vi "SIM Runge-Kutta embedded int (array).vi"(3 "Simulation data":T1={"continuous integrator"=enum."RK 1 (Euler)", "initial time"=0.1, "final time"=4.0, "step size"=600.0, "proposed step size"=1e-07, "max step size"=0.001, "min step size"=0.0, "discrete time step"=0.0, "max step ratio"=3.0, "Diag Eval Stage"=enum."Major Substep", "Substep Index"=0, "Timestep Index"=10.0, "simulation time"=0.0, "current timestep base"=0.01, "proposed step time"=0.0, "absolute tolerance"=0.0, "relative tolerance"=0.0, "step accepted?"=FALSE, "step complete?"=FALSE, "Halt?"=FALSE, "reset integrator?"=FALSE, "machine epsilon"=6.0, "min float"=0.0, "error"={"status"=FALSE, "code"=0, "source"=""}, "Method Order"=0, "Finished Late [i-1]"=FALSE, "Discrete step?"=FALSE, "NaN and Inf check?"=FALSE, "Final Timestep Index"=0.0, "(maj+disc)or(init)?"=FALSE, "Full Solver Reset"=TRUE, "Execution Mode"=0, "check vector sizes?"=FALSE, "solver handles zc?"=FALSE, "Simulation Registry"={"Current Idx"=0, "Node Tags"=[], "Node Headers"=[], "Node Data"=[], "Cont State data"={"inputs"=[], "outputs"=[], "reset"=[], "lower limits"=[], "upper limits"=[], "limit types"=[], "reset types"=[], "initial conditions"=[], "reset I.C."=[], "limited?"=[], "State Names"=[]}, "DiscreteInfo"={"tick period (sec)"=0.0, "time (ticks)"=0, "fire?"=[], "registry"={"period (sec)"=[], "skew (sec)"=[], "period (tick)"=[], "skew (tick)"=[]}, "discrete \nblocks?"=FALSE, "steps per tick"=0.0, "steps to tick"=0.0, "discrete \ntick?"=FALSE}, "Disc State data"={"Disc States"=[], "State Names"=[]}, "Registry Error"={"Error Block ID"=0, "code"=0}, "ZC Indices"=[]}, "variable step solver?"=FALSE, "First Substep?"=FALSE, "Continuous States?"=FALSE} {"Execution Mode" items=["Simulate to Completion", "Single Time-Step Simulation (Fixed Step Only)"]; "min float" format="%.1e"; "proposed step size" format="%.1e"; "proposed step time" format="%.1e"; "max step ratio" format="%.1e"; "min step size" format="%.1e"; "machine epsilon" format="%.1e"; "discrete time step" format="%.1e"; "max step size" format="%.1e"; "current timestep base" format="%.1e"; "final time" format="%.1e"; "simulation time" format="%.1e"; "relative tolerance" format="%.1e"; "absolute tolerance" format="%.1e"; "Substep Index" format="%.1e"; "step size" format="%.1e"; "initial time" format="%.1e"}) -> (1 "Simulation data out":T1={"continuous integrator"=enum."RK 1 (Euler)", "initial time"=0.1, "final time"=4.0, "step size"=600.0, "proposed step size"=1e-07, "max step size"=0.001, "min step size"=0.0, "discrete time step"=0.0, "max step ratio"=3.0, "Diag Eval Stage"=enum."Major Substep", "Substep Index"=0, "Timestep Index"=10.0, "simulation time"=0.0, "current timestep base"=0.01, "proposed step time"=0.0, "absolute tolerance"=0.0, "relative tolerance"=0.0, "step accepted?"=FALSE, "step complete?"=FALSE, "Halt?"=FALSE, "reset integrator?"=FALSE, "machine epsilon"=6.0, "min float"=0.0, "error"={"status"=FALSE, "code"=0, "source"=""}, "Method Order"=0, "Finished Late [i-1]"=FALSE, "Discrete step?"=FALSE, "NaN and Inf check?"=FALSE, "Final Timestep Index"=0.0, "(maj+disc)or(init)?"=FALSE, "Full Solver Reset"=TRUE, "Execution Mode"=0, "check vector sizes?"=FALSE, "solver handles zc?"=FALSE, "Simulation Registry"={"Current Idx"=0, "Node Tags"=[], "Node Headers"=[], "Node Data"=[], "Cont State data"={"inputs"=[], "outputs"=[], "reset"=[], "lower limits"=[], "upper limits"=[], "limit types"=[], "reset types"=[], "initial conditions"=[], "reset I.C."=[], "limited?"=[], "State Names"=[]}, "DiscreteInfo"={"tick period (sec)"=0.0, "time (ticks)"=0, "fire?"=[], "registry"={"period (sec)"=[], "skew (sec)"=[], "period (tick)"=[], "skew (tick)"=[]}, "discrete \nblocks?"=FALSE, "steps per tick"=0.0, "steps to tick"=0.0, "discrete \ntick?"=FALSE}, "Disc State data"={"Disc States"=[], "State Names"=[]}, "Registry Error"={"Error Block ID"=0, "code"=0}, "ZC Indices"=[]}, "variable step solver?"=FALSE, "First Substep?"=FALSE, "Continuous States?"=FALSE} {"Execution Mode" items=["Simulate to Completion", "Single Time-Step Simulation (Fixed Step Only)"]; "min float" format="%.1e"; "proposed step size" format="%.1e"; "proposed step time" format="%.1e"; "max step ratio" format="%.1e"; "min step size" format="%.1e"; "machine epsilon" format="%.1e"; "discrete time step" format="%.1e"; "max step size" format="%.1e"; "current timestep base" format="%.1e"; "final time" format="%.1e"; "simulation time" format="%.1e"; "relative tolerance" format="%.1e"; "absolute tolerance" format="%.1e"; "Substep Index" format="%.1e"; "step size" format="%.1e"; "initial time" format="%.1e"})   [LabVIEW 2010]
uses:
  SIM simulation data.ctl
  SIM integration method.ctl
  SIM diagram eval stage.ctl
  SIMSCR Execution Mode.ctl
  SIM Simulation Registry.ctl
  SIM Registry Node Header.ctl
  SIM Registry Node Record.ctl
  SIM trigger type.ctl
  SIM solver state data.ctl
  SIM limit type.ctl
  SIM discrete data.ctl
  SIM Discrete state data.ctl
  SIM Simulation Registry Error.ctl
  SIM limit signal (array).vi
panel:
  # "General Runge-Kutta integrator of order s.\n\nSolves the initial value problem \n\ny'(t) = f(t,y)\n\nby propogating the solution from y(t_n) to y(t_(n+1)), using the intermediate function evaluations k_i. The stepsize is defined as h = t_(n+1) - t_n.\n\nk_i = f( t_n + c_i h, y_n + h sum(j = 1 to s)(a_ij k_j) ) (1 <= i <= s)\n\ny_(n+1) = y_n + h sum(j = 1 to s)(a_(s-1)j k_j )\n\nNOTE This VI is paired with a time advancer that makes the simulation time appropriate for evaluating the k_i.\n\nNOTE This implementation assumes that c_0 = 0 and that\na_0j = 0 for a <= j <= s. The first row (all zeros) of the matrix a\nis omitted, and the last row of a stores the coefficients for the final output. Consequently, in the equation for k_i, a_ij should really read a_(i-1)j ."
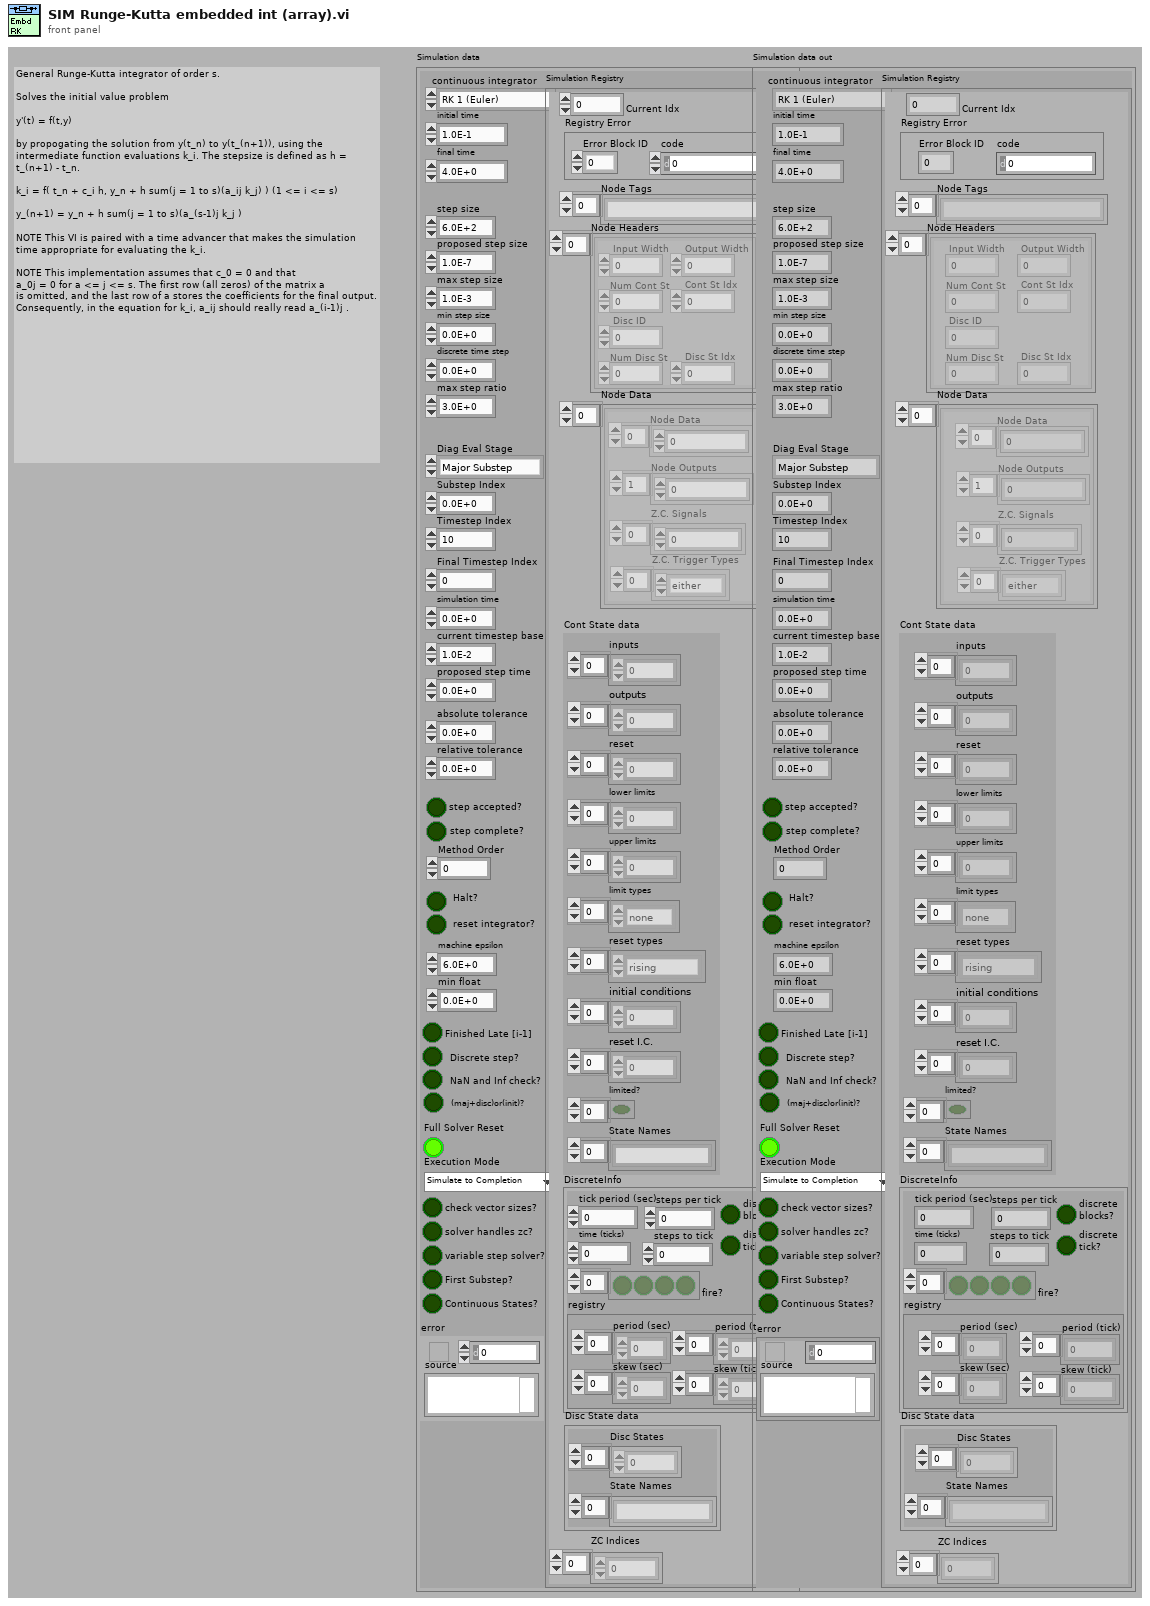
[diagram p1: front panel]
types:
  T1 = typedef "SIM simulation data.ctl" = cluster{"continuous integrator":T2, "initial time":dbl, "final time":dbl, "step size":dbl, "proposed step size":dbl, "max step size":dbl, "min step size":dbl, "discrete time step":dbl, "max step ratio":dbl, "Diag Eval Stage":T3, "Substep Index":i32, "Timestep Index":dbl, "simulation time":dbl, "current timestep base":dbl, "proposed step time":dbl, "absolute tolerance":dbl, "relative tolerance":dbl, "step accepted?":bool, "step complete?":bool, "Halt?":bool, "reset integrator?":bool, "machine epsilon":dbl, "min float":dbl, "error":errorcluster, "Method Order":u32, "Finished Late [i-1]":bool, "Discrete step?":bool, "NaN and Inf check?":bool, "Final Timestep Index":dbl, "(maj+disc)or(init)?":bool, "Full Solver Reset":bool, "Execution Mode":T4, "check vector sizes?":bool, "solver handles zc?":bool, "Simulation Registry":T5, "variable step solver?":bool, "First Substep?":bool, "Continuous States?":bool}
  T2 = typedef "SIM integration method.ctl" = enum16{"RK 1 (Euler)", "Linearizer", "State Query", "Trim Eval", "Adams", "RK 3", "RK 4", "RK 45", "BDF", "RK 2", "RK 23", "Rosenbrock", "Discrete States Only"}
  T3 = typedef "SIM diagram eval stage.ctl" = enum16{"Init", "Minor Substep", "Major Substep", "Final"}
  T4 = typedef "SIMSCR Execution Mode.ctl" = u16
  T5 = typedef "SIM Simulation Registry.ctl" = cluster{"Current Idx":i32, "Node Tags":string[], "Node Headers":T6[], "Node Data":T7[], "Cont State data":T9, "DiscreteInfo":T11, "Disc State data":T12, "Registry Error":T13, "ZC Indices":i32[]}
  T6 = typedef "SIM Registry Node Header.ctl" = cluster{"Input Width":i32, "Disc ID":i32, "Num Cont St":i32, "Cont St Idx":i32, "Num Disc St":i32, "Disc St Idx":i32, "Output Width":i32}
  T7 = typedef "SIM Registry Node Record.ctl" = cluster{"Node Data":dbl[], "Node Outputs":dbl[], "Z.C. Signals":dbl[], "Z.C. Trigger Types":T8[]}
  T8 = typedef "SIM trigger type.ctl" = enum16{"rising", "falling", "either", "none"}
  T9 = typedef "SIM solver state data.ctl" = cluster{"inputs":dbl[], "outputs":dbl[], "reset":dbl[], "lower limits":dbl[], "upper limits":dbl[], "limit types":T10[], "reset types":T8[], "initial conditions":dbl[], "reset I.C.":dbl[], "limited?":bool[], "State Names":string[]}
  T10 = typedef "SIM limit type.ctl" = enum16{"upper", "lower", "both", "none"}
  T11 = typedef "SIM discrete data.ctl" = cluster{"tick period (sec)":dbl, "time (ticks)":i32, "fire?":bool[], "registry":cluster{"period (sec)":dbl[], "skew (sec)":dbl[], "period (tick)":i32[], "skew (tick)":i32[]}, "discrete \nblocks?":bool, "steps per tick":dbl, "steps to tick":dbl, "discrete \ntick?":bool}
  T12 = typedef "SIM Discrete state data.ctl" = cluster{"Disc States":dbl[], "State Names":string[]}
  T13 = typedef "SIM Simulation Registry Error.ctl" = cluster{"Error Block ID":i32, "code":i32}
  T14 = typedef "SIM Runga-Kutte data - variable step.ctl" = cluster{"weighting coefficients":dbl[][], "time step fractions":dbl[], "Number of sub steps":i32, "error coefficients":dbl[], "error order":i32}
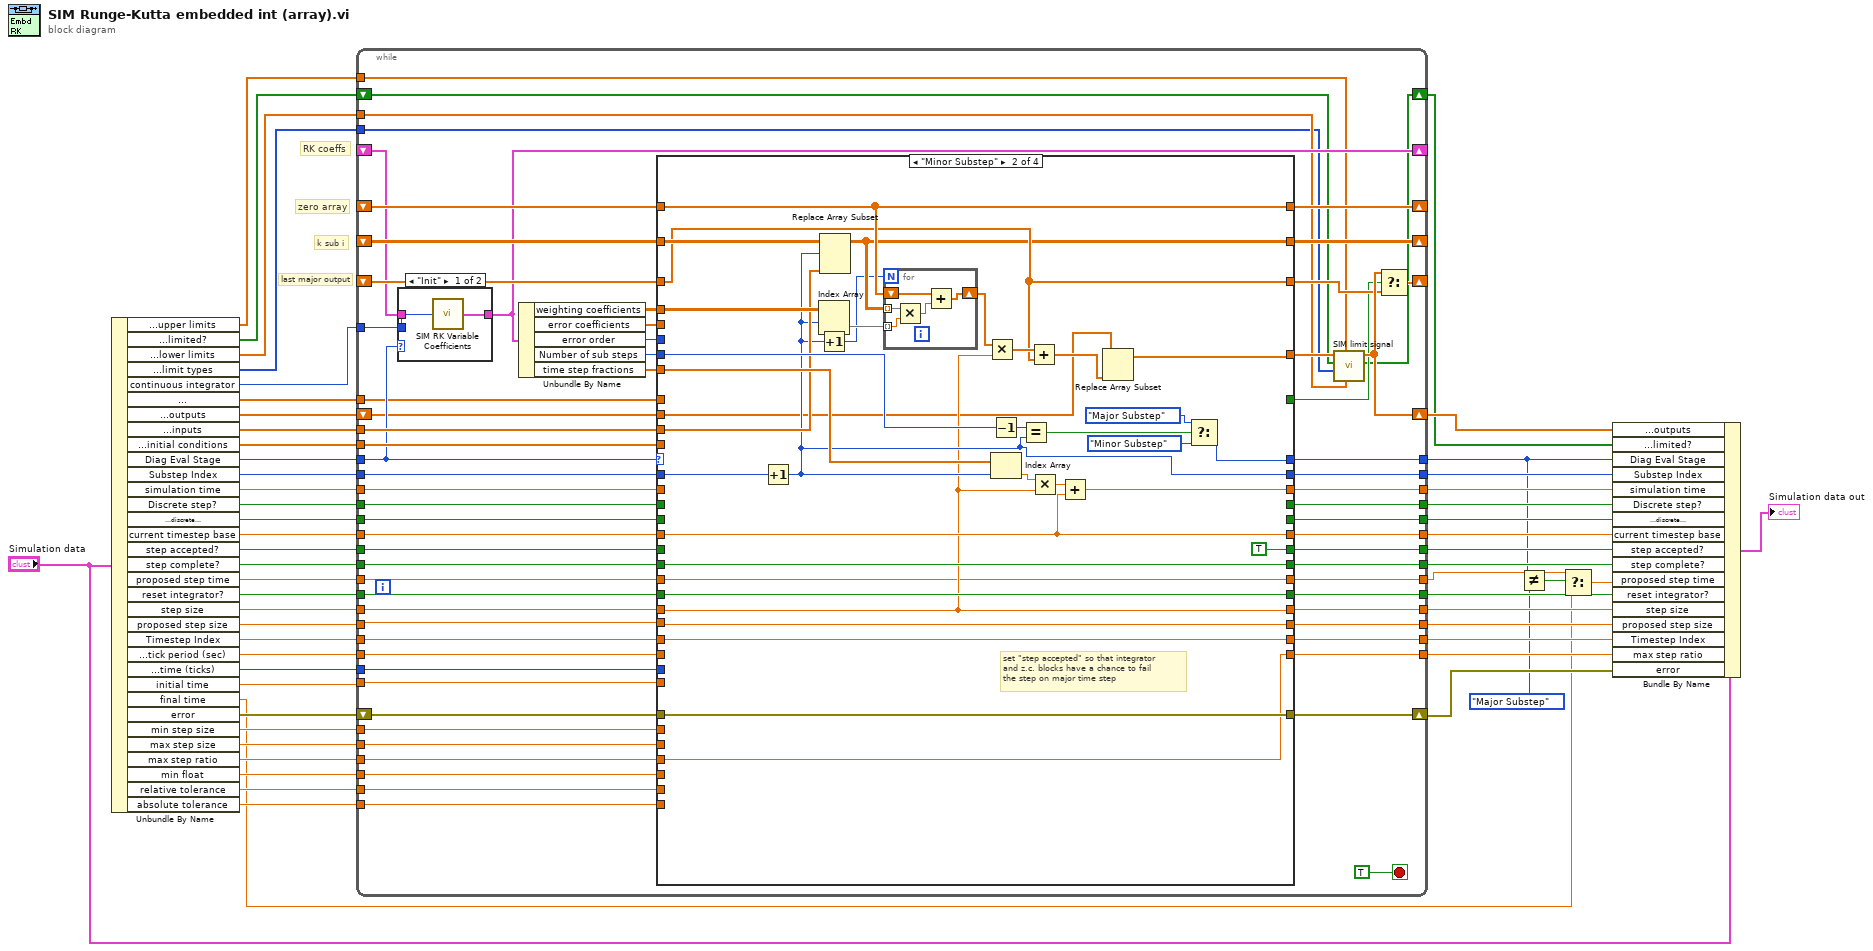
[diagram p0: block diagram]
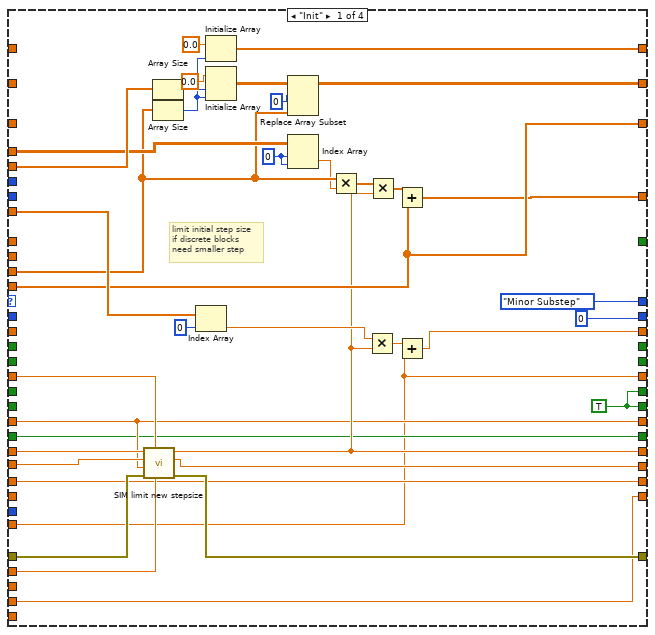
[diagram p3: hidden frame]
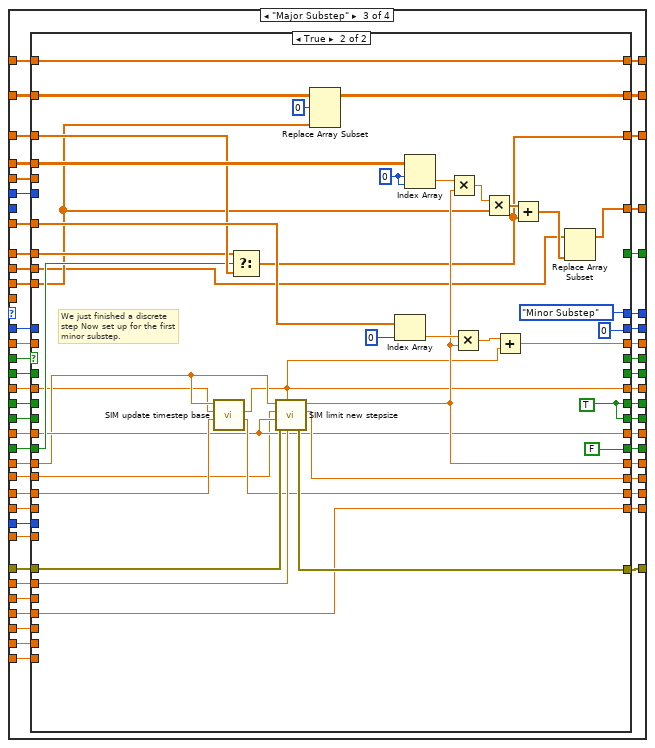
[diagram p4: hidden frame]
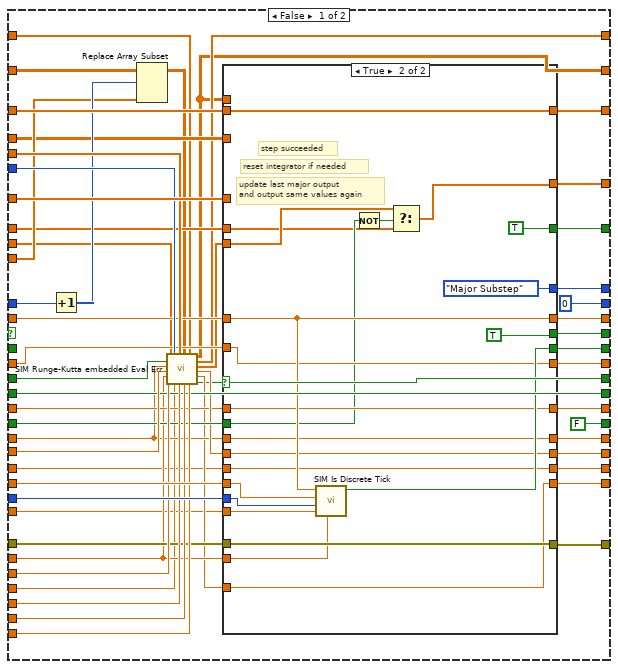
[diagram p5: hidden frame]
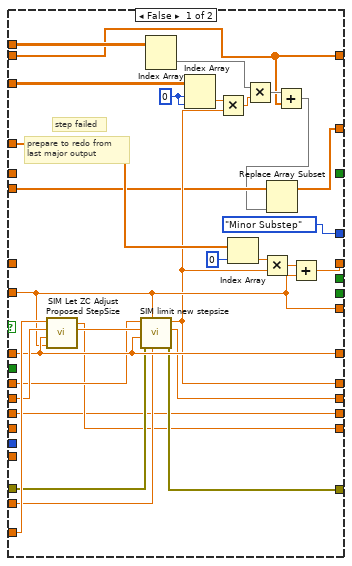
[diagram p6: hidden frame]
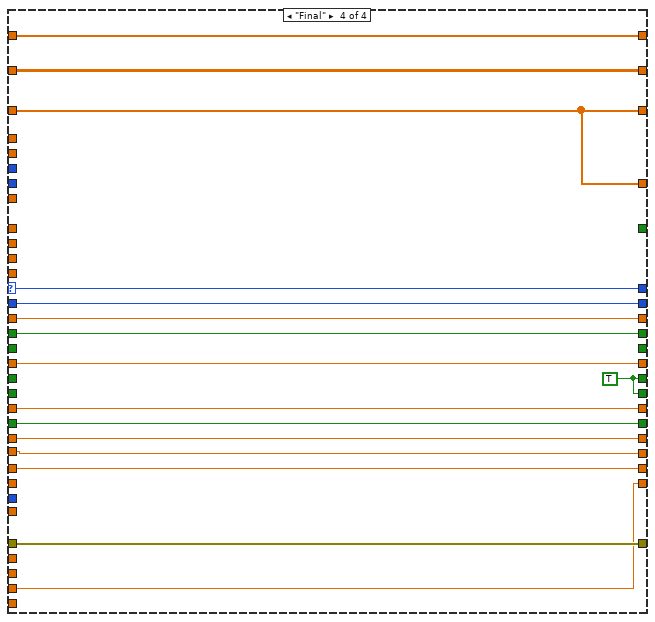
[diagram p7: hidden frame]
diagram:
  # "RK coeffs"
  # "last major output"
  # "k sub i"
  # "zero array"
  n1 = Unbundle By Name("Simulation data") -> ("Simulation Registry.Cont State data.upper limits"=w13:dbl[], "Simulation Registry.Cont State data.limited?"=w10:bool[], "Simulation Registry.Cont State data.lower limits"=w12:dbl[], "Simulation Registry.Cont State data.limit types"=w11:T10[], "continuous integrator"=w32:T2, "Simulation Registry.Cont State data.reset I.C."=w16:dbl[], "Simulation Registry.Cont State data.outputs"=w15:dbl[], "Simulation Registry.Cont State data.inputs"=w42:dbl[], "Simulation Registry.Cont State data.initial conditions"=w41:dbl[], "Diag Eval Stage"=w43:T3, "Substep Index"=w44:i32, "simulation time"=w38:dbl, "Discrete step?"=w8:bool, "Simulation Registry.DiscreteInfo.discrete \ntick?"=w7:bool, "current timestep base"=w36:dbl, "step accepted?"=w17:bool, "step complete?"=w27:bool, "proposed step time"=w35:dbl, "reset integrator?"=w29:bool, "step size"=w31:dbl, "proposed step size"=w30:dbl, "Timestep Index"=w23:dbl, "Simulation Registry.DiscreteInfo.tick period (sec)"=w40:dbl, "Simulation Registry.DiscreteInfo.time (ticks)"=w39:i32, "initial time"=w37:dbl, "final time"=w2:dbl, "error"=w28:errorcluster, "min step size"=w24:dbl, "max step size"=w22:dbl, "max step ratio"=w21:dbl, "min float"=w20:dbl, "relative tolerance"=w19:dbl, "absolute tolerance"=w18:dbl)
  n2 = while {
    shift-right: [w111] -> _
    shift-left: _ -> [w119]
    tunnel: w11 -> [w102]
    tunnel: w12 -> [w103]
    tunnel: w13 -> [w104]
    shift-right: [w110] -> _
    shift-left: _ -> [w115]
    shift-right: [w117] -> _
    shift-left: _ -> [w118]
    shift-right: [w106] -> _
    shift-left: _ -> [w105]
    tunnel: [w101] -> w5
    tunnel: [w100] -> w53
    tunnel: [w99] -> w52
    tunnel: [w98] -> w51
    tunnel: [w97] -> w50
    tunnel: [w96] -> w49
    tunnel: [w95] -> w48
    tunnel: [w94] -> w47
    tunnel: [w93] -> w3
    tunnel: [w92] -> w46
    tunnel: w44 -> [w91]
    tunnel: w43 -> [w88]
    tunnel: w42 -> [w90]
    tunnel: w41 -> [w89]
    tunnel: w8 -> [w87]
    tunnel: w40 -> [w86]
    tunnel: w39 -> [w85]
    tunnel: w38 -> [w84]
    tunnel: w37 -> [w82]
    tunnel: w36 -> [w81]
    tunnel: w24 -> [w78]
    tunnel: w35 -> [w77]
    tunnel: [w76] -> w34
    tunnel: [w75] -> w33
    tunnel: w32 -> [w74]
    tunnel: w31 -> [w73]
    tunnel: w30 -> [w72]
    tunnel: w29 -> [w71]
    tunnel: w27 -> [w70]
    tunnel: w23 -> [w69]
    tunnel: [w68] -> w25
    tunnel: w22 -> [w67]
    tunnel: w21 -> [w66]
    tunnel: w20 -> [w65]
    tunnel: w19 -> [w64]
    tunnel: w18 -> [w63]
    tunnel: w17 -> [w62]
    tunnel: w16 -> [w61]
    tunnel: [w59] -> w14
    shift-right: [w57] -> w9
    shift-left: w10 -> [w58]
    shift-right: [w109] -> w55
    shift-left: w15 -> [w60]
    shift-right: [w79] -> w26
    shift-left: w28 -> [w80]
    tunnel: w7 -> [w56]
    stop <- TRUE stop-if-true
    n3 = case shown="\"Init\"" w88 {
      tunnel: [w123 w124] -> w106
      tunnel: w105 -> [_ w124]
      tunnel: w74 -> [w122 _]
      frame "Init" {
        n4 = call "SIM RK Variable Coefficients.vi"("continuous integrator"=w122) -> ("Runga-Kutte data"=w123:T14)
      }
      frame Default {
      }
    }
    n5 = Unbundle By Name(w106) -> ("weighting coefficients"=w83:dbl[][], "error coefficients"=w114:dbl[], "error order"=w113:i32, "Number of sub steps"=w121:i32, "time step fractions"=w120:dbl[])
    n6 = case shown="\"Minor Substep\"" w88 {
      selector: w88 -> [_ _ _ w412]
      tunnel: [0 w177 w254 w411] -> w100
      tunnel: w120 -> [w161 w197 w252 _]
      tunnel: [w157 w194 w253 w408] -> w99
      tunnel: [SIM_diagram_eval_stage."Minor Substep" ("Diagram Eval Stage") w190 w251 w412] -> w101
      tunnel: w121 -> [_ w193 _ _]
      tunnel: w119 -> [_ w187 w244 w415]
      tunnel: w118 -> [_ w183 w250 w414]
      tunnel: w89 -> [w143 _ _ _]
      tunnel: [w147 w180 w240 w415] -> w111
      tunnel: [w151 w183 w238 w414] -> w117
      tunnel: w114 -> [w150 _ w248 _]
      tunnel: w115 -> [_ w181 w247 w413]
      tunnel: [w143 w181 w246 w413] -> w108
      tunnel: w91 -> [_ w178 w245 w411]
      tunnel: w113 -> [_ _ w249 _]
      tunnel: w90 -> [w127 w179 w243 _]
      tunnel: w83 -> [w141 w186 w241 _]
      tunnel: [w142 w165 w242 w413] -> w112
      tunnel: [_ _ w239 _] -> w107
      tunnel: w87 -> [_ _ w237 w410]
      tunnel: [_ _ w236 w410] -> w98
      tunnel: w85 -> [_ _ w235 _]
      tunnel: w86 -> [_ _ w234 _]
      tunnel: [_ _ w233 _] -> w97
      tunnel: [w125 w174 w216 w407] -> w96
      tunnel: [w140 TRUE ("step accepted?") w231 w409] -> w95
      tunnel: [w140 w173 w230 w409] -> w94
      tunnel: [w131 w163 w217 w406] -> w93
      tunnel: [w130 w172 w232 w405] -> w92
      tunnel: w84 -> [_ _ w207 w408]
      tunnel: w73 -> [w134 w171 w209 w404]
      tunnel: w82 -> [w125 _ w203 _]
      tunnel: w81 -> [w139 w174 w227 w407]
      tunnel: w80 -> [w138 w169 w221 w402]
      tunnel: [w137 w169 w222 w402] -> w79
      tunnel: w78 -> [w136 _ w223 _]
      tunnel: w72 -> [w135 w170 w225 w403]
      tunnel: w77 -> [w131 w163 w224 w406]
      tunnel: [w133 w171 w219 w404] -> w76
      tunnel: [w132 w170 w220 w403] -> w75
      tunnel: w71 -> [w130 w172 w228 w405]
      tunnel: w70 -> [_ w173 w206 _]
      tunnel: w61 -> [_ _ w229 _]
      tunnel: w69 -> [w129 w168 w226 w400]
      tunnel: [w129 w168 w218 w400] -> w68
      tunnel: w67 -> [_ _ w215 _]
      tunnel: w66 -> [w128 w167 w214 w401]
      tunnel: w65 -> [_ _ w213 _]
      tunnel: w64 -> [_ _ w212 _]
      tunnel: w63 -> [_ _ w211 _]
      tunnel: w62 -> [_ _ w210 _]
      tunnel: w60 -> [_ w164 w208 _]
      tunnel: [w128 w167 w205 w401] -> w59
      tunnel: w56 -> [_ _ w204 _]
      frame "Init" {
        w146 = 0 ("index (row)")
        w140 = TRUE ("step accepted?")
        # "limit initial step size\nif discrete blocks\nneed smaller step"
        n7 = call "SIM limit new stepsize.vi"("min step size"=w136, "current timestep base"=w139, "error"=w138, "proposed step time"=w131, "proposed step size"=w135, "step size"=w134) -> ("error out"=w137:errorcluster, "proposed step size"=w132:dbl, "step size"=w133:dbl)  [unwired: 1 in, 2 out]
        n8 = Array Size(array=w150) -> (size(s)=w155:i32)
        n9 = Array Size(array=w127) -> (size(s)=w152:i32)
        n10 = Index Array(array=w161, index=0) -> (element=w159:dbl)
        n11 = Initialize Array(0.0 ("element"), w152) -> (w151:dbl[])
        n12 = Initialize Array(0.0 ("element"), w155, w152) -> (w149:dbl[][])
        n13 = Replace Array Subset(array=w149, new element=w127, index (row)=0) -> (w147:dbl[][])  [unwired: 1 in]
        n14 = Index Array(array=w141, index (row)=w146, index (col)=w146) -> (element=w126:dbl)
        n15 = Multiply(x=w127, y=w126) -> (x*y=w145:dbl[])
        n16 = Multiply(x=w159, y=w133) -> (x*y=w158:dbl)
        n17 = Multiply(x=w145, y=w133) -> (x*y=w144:dbl[])
        n18 = Add(x=w144, y=w143) -> (x+y=w142:dbl[])
        n19 = Add(x=w158, y=w125) -> (x+y=w157:dbl)
      }
      frame "Minor Substep" {
        # "set \"step accepted\" so that integrator\nand z.c. blocks have a chance to fail \nthe step on major time step"
        n20 = Increment(x=w178) -> (x+1=w177:i32)
        n21 = Index Array(array=w186, index (row)=w177) -> (element=w184:dbl[])  [unwired: 1 in]
        n22 = Increment(x=w177) -> (x+1=w176:i32)
        n23 = Replace Array Subset(array=w187, new element=w179, index (row)=w177) -> (w180:dbl[][])  [unwired: 1 in]
        n24 = for {
          N: w176 -> [_]
          tunnel: w180 -> [w202] mode=indexing
          tunnel: w184 -> [w201] mode=indexing
          shift-right: [w199] -> w185
          shift-left: w183 -> [w198]
          n25 = Multiply(x=w202, y=w201) -> (x*y=w200:dbl[])
          n26 = Add(x=w198, y=w200) -> (x+y=w199:dbl[])
        }
        n27 = Multiply(x=w185, y=w171) -> (x*y=w182:dbl[])
        n28 = Decrement(x=w193) -> (x-1=w192:i32)
        n29 = Index Array(array=w197, index=w177) -> (element=w196:dbl)
        n30 = Equal?(x=w192, y=w177) -> (x = y?=w191:bool)
        n31 = Add(x=w182, y=w181) -> (x+y=w166:dbl[])
        n32 = Multiply(x=w196, y=w171) -> (x*y=w195:dbl)
        n33 = Add(x=w195, y=w174) -> (x+y=w194:dbl)
        n34 = Replace Array Subset(array=w164, new element=w166) -> (w165:dbl[])  [unwired: 1 in]
        n35 = Select(t=SIM_diagram_eval_stage."Major Substep" ("Diagram Eval Stage"), s=w191, f=SIM_diagram_eval_stage."Minor Substep" ("Diagram Eval Stage")) -> (s? t:f=w190:T3)
      }
      frame "Major Substep" {
        n36 = case shown="True" w237 {
          tunnel: [0 ("Substep Index") 0 ("Substep Index")] -> w254
          tunnel: [w307 w365] -> w253
          tunnel: w252 -> [w306 w385]
          tunnel: [w305 SIM_diagram_eval_stage."Minor Substep" ("Diagram Eval Stage")] -> w251
          tunnel: w250 -> [w262 w389]
          tunnel: w249 -> [w304 _]
          tunnel: w248 -> [w303 _]
          tunnel: w247 -> [w302 w384]
          tunnel: [w301 w370] -> w246
          tunnel: w245 -> [w300 _]
          tunnel: w244 -> [w299 w390]
          tunnel: w243 -> [w297 w372]
          tunnel: [w296 w366] -> w242
          tunnel: w241 -> [w295 w391]
          tunnel: [w257 w388] -> w240
          tunnel: [w294 _] -> w239
          tunnel: [w261 w389] -> w238
          tunnel: [w293 _] -> w236
          tunnel: w235 -> [w292 _]
          tunnel: w234 -> [w291 _]
          tunnel: [w290 _] -> w233
          tunnel: [FALSE ("reset integrator?") FALSE ("reset integrator?")] -> w232
          tunnel: [w260 w383] -> w231
          tunnel: [w280 w383] -> w230
          tunnel: w229 -> [w283 w382]
          tunnel: w228 -> [w282 w381]
          tunnel: w227 -> [w278 w362]
          tunnel: w226 -> [w265 w379]
          tunnel: w225 -> [w284 w363]
          tunnel: w224 -> [w275 w371]
          tunnel: w223 -> [w271 w378]
          tunnel: [w272 w377] -> w222
          tunnel: w221 -> [w273 w376]
          tunnel: [w276 w375] -> w220
          tunnel: [w266 w374] -> w219
          tunnel: [w264 w373] -> w218
          tunnel: [w274 w371] -> w217
          tunnel: [w267 w361] -> w216
          tunnel: w215 -> [w288 _]
          tunnel: w214 -> [w269 w369]
          tunnel: w213 -> [w287 _]
          tunnel: w212 -> [w286 _]
          tunnel: w211 -> [w285 _]
          tunnel: w210 -> [w279 _]
          tunnel: w209 -> [w270 w364]
          tunnel: w208 -> [w259 w367]
          tunnel: w207 -> [w281 _]
          tunnel: w206 -> [w280 _]
          tunnel: [w256 w369] -> w205
          tunnel: w204 -> [_ _]
          tunnel: w203 -> [w255 _]
          frame False {
            n37 = Increment(x=w300) -> (x+1=w298:i32)
            n38 = Replace Array Subset(array=w299, new element=w297, index (row)=w298) -> (w263:dbl[][])  [unwired: 1 in]
            n39 = call "SIM Runge-Kutta embedded Eval Err.vi"("outputs"=w259, "step accepted?"=w279, "step size"=w270, "proposed step size"=w284, "min step size"=w271, "max step size"=w288, "error order"=w304, "max step ratio"=w269, "error coefficients"=w303, "min float"=w287, "k sub i"=w263, "relative tolerance"=w286, "Zero Array"=w262, "absolute tolerance"=w285) -> ("k sub i out"=w257:dbl[][], "Zero Array Out"=w261:dbl[], "outputs out"=w258:dbl[], "proposed step size out"=w277:dbl, "new step size ratio"=w268:dbl, "step accepted? out"=w260:bool)
            n40 = case shown="True" w260 {
              tunnel: [w338 w353] -> w307
              tunnel: w306 -> [w337 _]
              tunnel: [SIM_diagram_eval_stage."Minor Substep" ("Diagram Eval Stage") SIM_diagram_eval_stage."Major Substep" ("Diagram Eval Stage")] -> w305
              tunnel: w302 -> [w309 w359]
              tunnel: [w309 w359] -> w301
              tunnel: [w313 w357] -> w296
              tunnel: w257 -> [w330 _]
              tunnel: w295 -> [w331 _]
              tunnel: [_ TRUE] -> w294
              tunnel: [_ TRUE] -> w293
              tunnel: w292 -> [_ w355]
              tunnel: w291 -> [_ w350]
              tunnel: [_ w354] -> w290
              tunnel: w283 -> [_ w341]
              tunnel: w282 -> [_ w343]
              tunnel: w258 -> [w315 w342]
              tunnel: w281 -> [_ w353]
              tunnel: w268 -> [w326 w348]
              tunnel: w278 -> [w317 w347]
              tunnel: w277 -> [w325 w351]
              tunnel: [w311 w351] -> w276
              tunnel: w275 -> [w323 w352]
              tunnel: [w323 w352] -> w274
              tunnel: w273 -> [w322 w349]
              tunnel: [w321 w349] -> w272
              tunnel: w271 -> [w320 w339]
              tunnel: w270 -> [w319 w345]
              tunnel: [w318 w348] -> w256
              tunnel: [w317 w347] -> w267
              tunnel: [w316 w345] -> w266
              tunnel: w265 -> [w310 w346]
              tunnel: [w310 w346] -> w264
              tunnel: w255 -> [_ w340]
              frame False {
                w333 = 0 ("index (row)")
                # "step failed"
                # "prepare to redo from\nlast major output"
                n41 = call "SIM Let ZC Adjust Proposed StepSize.vi"("current timestep base"=w317, "proposed step time"=w323, "proposed step size"=w325, "max step ratio"=w326) -> ("proposed step size out"=w324:dbl, "max step ratio out"=w318:dbl)  [unwired: 2 out]
                n42 = call "SIM limit new stepsize.vi"("min step size"=w320, "current timestep base"=w317, "error"=w322, "proposed step time"=w323, "proposed step size"=w324, "step size"=w319) -> ("error out"=w321:errorcluster, "proposed step size"=w311:dbl, "step size"=w316:dbl)  [unwired: 1 in, 2 out]
                n43 = Index Array(array=w330) -> (element=w327:dbl[])  [unwired: 2 in]
                n44 = Index Array(array=w331, index (row)=w333, index (col)=w333) -> (element=w329:dbl)
                n45 = Multiply(x=w329, y=w316) -> (x*y=w328:dbl)
                n46 = Index Array(array=w337, index=0) -> (element=w336:dbl)
                n47 = Multiply(x=w327, y=w328) -> (x*y=w332:dbl[])
                n48 = Multiply(x=w336, y=w316) -> (x*y=w334:dbl)
                n49 = Add(x=w332, y=w309) -> (x+y=w314:dbl[])
                n50 = Replace Array Subset(array=w315, new element=w314) -> (w313:dbl[])  [unwired: 1 in]
                n51 = Add(x=w334, y=w317) -> (x+y=w338:dbl)
              }
              frame True {
                # "reset integrator if needed"
                # "step succeeded"
                # "update last major output\nand output same values again"
                n52 = call "SIM Is Discrete Tick.vi"("min step size"=w339, "initial time"=w340, "time (ticks)"=w355, "tick period (sec)"=w350, "simulation time"=w353) -> ("Discrete Tick?"=w354:bool)  [unwired: 6 out]
                n53 = Not(x=w343) -> (.not. x?=w344:bool)
                n54 = Select(t=w342, s=w344, f=w341) -> (s? t:f=w357:dbl[])
              }
            }
          }
          frame True {
            w395 = 0 ("index (row)")
            w383 = TRUE ("step complete?")
            # "We just finished a discrete\nstep Now set up for the first\nminor substep."
            n55 = call "SIM update timestep base.vi"("Timestep Index"=w379, "current timestep base"=w362, "step size"=w364) -> ("Timestep Index out"=w373:dbl, "current timestep base out"=w361:dbl)  [unwired: 1 in, 2 out]
            n56 = Select(t=w382, s=w381, f=w384) -> (s? t:f=w370:dbl[])
            n57 = call "SIM limit new stepsize.vi"("min step size"=w378, "current timestep base"=w361, "error"=w376, "proposed step time"=w371, "proposed step size"=w363, "step size"=w364) -> ("error out"=w377:errorcluster, "proposed step size"=w375:dbl, "step size"=w374:dbl)  [unwired: 1 in, 2 out]
            n58 = Replace Array Subset(array=w390, new element=w372, index (row)=0) -> (w388:dbl[][])  [unwired: 1 in]
            n59 = Index Array(array=w385, index=0 ("Substep Index")) -> (element=w398:dbl)
            n60 = Index Array(array=w391, index (row)=w395, index (col)=w395) -> (element=w394:dbl)
            n61 = Multiply(x=w394, y=w374) -> (x*y=w393:dbl)
            n62 = Multiply(x=w398, y=w374) -> (x*y=w399:dbl)
            n63 = Multiply(x=w393, y=w372) -> (x*y=w392:dbl[])
            n64 = Add(x=w399, y=w361) -> (x+y=w365:dbl)
            n65 = Add(x=w392, y=w370) -> (x+y=w368:dbl[])
            n66 = Replace Array Subset(array=w367, new element=w368) -> (w366:dbl[])  [unwired: 1 in]
          }
        }
      }
      frame "Final" {
        w409 = TRUE ("step accepted?")
      }
    }
    n67 = call-poly "SIM limit signal.vi"("lower limits"=w103, "upper limits"=w104, "limit types"=w102, "limited? in"=w58, "inputs"=w112) -> ("limited? out"=w57:bool[], "outputs"=w109:dbl[])  [unwired: 1 in, 4 out]
    n68 = Select(t=w109, s=w107, f=w108) -> (s? t:f=w110:dbl[])
  }
  n69 = Not Equal?(x=w5, y=SIM_diagram_eval_stage."Major Substep") -> (x != y?=w4:bool)
  n70 = Select(t=w3, s=w4, f=w2) -> (s? t:f=w1:dbl)
  n71 = Bundle By Name(cluster="Simulation data", "Simulation Registry.Cont State data.outputs"=w55, "Simulation Registry.Cont State data.limited?"=w9, "Diag Eval Stage"=w5, "Substep Index"=w53, "simulation time"=w52, "Discrete step?"=w51, "Simulation Registry.DiscreteInfo.discrete \ntick?"=w50, "current timestep base"=w49, "step accepted?"=w48, "step complete?"=w47, "proposed step time"=w1, "reset integrator?"=w46, "step size"=w34, "proposed step size"=w33, "Timestep Index"=w25, "max step ratio"=w14, "error"=w26) -> (→"Simulation data out":T1)
